vi "Lab Panel V5.23.vi"() -> ()   [LabVIEW 2013] (continued)
                n1762 = property on="SELECT LAB01-1" class="RadioBtnsControl (strict)"("DisabledEnum"=w3329) -> ()  [unwired: 2 in, 2 out]
                n1763 = property on="SELECT LAB01-2" class="RadioBtnsControl (strict)"("DisabledEnum"=w3328) -> ()  [unwired: 2 in, 2 out]
                n1764 = Not(x=w3338) -> (.not. x?=w3339:bool)
                n1765 = property on="RESULT LAB01-1" class="Bool (strict)"("Visible"=w3339) -> ()  [unwired: 2 in, 2 out]
                n1766 = Not(x=w3333) -> (.not. x?=w3337:bool)
                n1767 = Not(x=w3332) -> (.not. x?=w3336:bool)
                n1768 = Not(x=w3330) -> (.not. x?=w3335:bool)
                n1769 = property on="RESULT LAB01-2" class="Bool (strict)"("Visible"=w3337) -> ()  [unwired: 2 in, 2 out]
                n1770 = Not(x=w3331) -> (.not. x?=w3334:bool)
                n1771 = property on="RESULT LAB02-1" class="Bool (strict)"("Visible"=w3336) -> ()  [unwired: 2 in, 2 out]
                n1772 = property on="RESULT LAB02-2" class="Bool (strict)"("Visible"=w3335) -> ()  [unwired: 2 in, 2 out]
                n1773 = property on="RESULT LAB03-1" class="Bool (strict)"("Visible"=w3334) -> ()  [unwired: 2 in, 2 out]
                n1774 = property on="SET LAB01-1" class="Clust (strict)"("DisabledEnum"=w3329) -> ()  [unwired: 2 in, 2 out]
                n1775 = property on="SET LAB01-2" class="Clust (strict)"("DisabledEnum"=w3328) -> ()  [unwired: 2 in, 2 out]
                n1776 = property on="SET LAB02-1" class="Clust (strict)"("DisabledEnum"=w3327) -> ()  [unwired: 2 in, 2 out]
                n1777 = property on="SET LAB02-2" class="Clust (strict)"("DisabledEnum"=w3326) -> ()  [unwired: 2 in, 2 out]
                n1778 = property on="SET LAB03-1" class="Clust (strict)"("DisabledEnum"=w3325) -> ()  [unwired: 2 in, 2 out]
                n1779 = property on="O/I  LAB01-1" class="Bool (strict)"("DisabledEnum"=w3329) -> ()  [unwired: 2 in, 2 out]
                n1780 = property on="O/I  LAB01-2" class="Bool (strict)"("DisabledEnum"=w3328) -> ()  [unwired: 2 in, 2 out]
                n1781 = property on="O/I  LAB02-1" class="Bool (strict)"("DisabledEnum"=w3327) -> ()  [unwired: 2 in, 2 out]
                n1782 = property on="O/I  LAB02-2" class="Bool (strict)"("DisabledEnum"=w3326) -> ()  [unwired: 2 in, 2 out]
                n1783 = property on="O/I  LAB03-1" class="Bool (strict)"("DisabledEnum"=w3325) -> ()  [unwired: 2 in, 2 out]
              }
              frame #1 {
                n1784 = Select(t=2, s=w3359, f=0) -> (s? t:f=w3350:i32)
                n1785 = Select(t=2, s=w3358, f=0) -> (s? t:f=w3351:i32)
                n1786 = Select(t=2, s=w3355, f=0) -> (s? t:f=w3354:i32)
                n1787 = Select(t=2, s=w3356, f=0) -> (s? t:f=w3353:i32)
                n1788 = Select(t=2, s=w3357, f=0) -> (s? t:f=w3352:i32)
                n1789 = property on="SELECT LAB05-2" class="RadioBtnsControl (strict)"("DisabledEnum"=w3350) -> ()  [unwired: 2 in, 2 out]
                n1790 = property on="SELECT LAB05-1" class="RadioBtnsControl (strict)"("DisabledEnum"=w3351) -> ()  [unwired: 2 in, 2 out]
                n1791 = property on="SELECT LAB03-2" class="RadioBtnsControl (strict)"("DisabledEnum"=w3354) -> ()  [unwired: 2 in, 2 out]
                n1792 = property on="SELECT LAB04-1" class="RadioBtnsControl (strict)"("DisabledEnum"=w3353) -> ()  [unwired: 2 in, 2 out]
                n1793 = property on="SELECT LAB04-2" class="RadioBtnsControl (strict)"("DisabledEnum"=w3352) -> ()  [unwired: 2 in, 2 out]
                n1794 = property on="SET LAB05-2" class="Clust (strict)"("DisabledEnum"=w3350) -> ()  [unwired: 2 in, 2 out]
                n1795 = property on="SET LAB05-1" class="Clust (strict)"("DisabledEnum"=w3351) -> ()  [unwired: 2 in, 2 out]
                n1796 = property on="SET LAB03-2" class="Clust (strict)"("DisabledEnum"=w3354) -> ()  [unwired: 2 in, 2 out]
                n1797 = property on="SET LAB04-1" class="Clust (strict)"("DisabledEnum"=w3353) -> ()  [unwired: 2 in, 2 out]
                n1798 = property on="SET LAB04-2" class="Clust (strict)"("DisabledEnum"=w3352) -> ()  [unwired: 2 in, 2 out]
                n1799 = property on="O/I  LAB05-2" class="Bool (strict)"("DisabledEnum"=w3350) -> ()  [unwired: 2 in, 2 out]
                n1800 = property on="O/I  LAB05-1" class="Bool (strict)"("DisabledEnum"=w3351) -> ()  [unwired: 2 in, 2 out]
                n1801 = property on="O/I  LAB04-1" class="Bool (strict)"("DisabledEnum"=w3353) -> ()  [unwired: 2 in, 2 out]
                n1802 = property on="O/I  LAB04-2" class="Bool (strict)"("DisabledEnum"=w3352) -> ()  [unwired: 2 in, 2 out]
                n1803 = property on="O/I  LAB03-2" class="Bool (strict)"("DisabledEnum"=w3354) -> ()  [unwired: 2 in, 2 out]
                n1804 = Not(x=w3359) -> (.not. x?=w3360:bool)
                n1805 = Not(x=w3358) -> (.not. x?=w3361:bool)
                n1806 = Not(x=w3357) -> (.not. x?=w3362:bool)
                n1807 = property on="RESULT LAB05-2" class="Bool (strict)"("Visible"=w3360) -> ()  [unwired: 2 in, 2 out]
                n1808 = property on="RESULT LAB05-1" class="Bool (strict)"("Visible"=w3361) -> ()  [unwired: 2 in, 2 out]
                n1809 = Not(x=w3356) -> (.not. x?=w3363:bool)
                n1810 = property on="RESULT LAB04-2" class="Bool (strict)"("Visible"=w3362) -> ()  [unwired: 2 in, 2 out]
                n1811 = Not(x=w3355) -> (.not. x?=w3364:bool)
                n1812 = property on="RESULT LAB04-1" class="Bool (strict)"("Visible"=w3363) -> ()  [unwired: 2 in, 2 out]
                n1813 = property on="RESULT LAB03-2" class="Bool (strict)"("Visible"=w3364) -> ()  [unwired: 2 in, 2 out]
              }
              frame #2 {
                # "disable calibrate if any test running"
                n1814 = Or(x=w3387, y=w3386) -> (x .or. y?=w3380:bool)
                n1815 = Or(x=w3389, y=w3388) -> (x .or. y?=w3382:bool)
                n1816 = Or(x=w3393, y=w3392) -> (x .or. y?=w3384:bool)
                n1817 = Or(x=w3391, y=w3390) -> (x .or. y?=w3383:bool)
                n1818 = Or(x=w3395, y=w3394) -> (x .or. y?=w3385:bool)
                n1819 = Or(x=w3383, y=w3382) -> (x .or. y?=w3381:bool)
                n1820 = Or(x=w3385, y=w3384) -> (x .or. y?=w3379:bool)
                n1821 = Or(x=w3381, y=w3380) -> (x .or. y?=w3378:bool)
                n1822 = Or(x=w3379, y=w3378) -> (x .or. y?=w3377:bool)
                n1823 = case shown="False" w3377 {
                  tunnel: [0 2] -> w3376
                  frame False {
                  }
                  frame True {
                  }
                }
                n1824 = property on="JIG TEST" class="Clust (strict)"("DisabledEnum"=w3376) -> ()  [unwired: 2 in, 2 out]
                n1825 = property on="Network Directory" class="Path"("DisabledEnum"=w3376) -> ()  [unwired: 2 in, 2 out]
                n1826 = property on="MAIL SETTINGS" class="Clust (strict)"("DisabledEnum"=w3376) -> ()  [unwired: 2 in, 2 out]
                n1827 = property on="SET (cal)" class="Bool (strict)"("DisabledEnum"=w3376) -> ()  [unwired: 2 in, 2 out]
                n1828 = property on="ADMIN" class="Bool (strict)"("DisabledEnum"=0) -> ()  [unwired: 2 in, 2 out]
              }
            }
          }
          frame #8 {
            # "drive jigs"
            n1829 = stacked-sequence {
              frame #0 {
                # "jig on"
                n1830 = local read "jig cycle"() -> (w3403:dbl)
                n1831 = property on="JIG TEST" class="Clust (strict)"() -> ("DisabledEnum"=w3400:T16)  [unwired: 2 in, 2 out]
                n1832 = Equal?(x=w3400, y=2) -> (x = y?=w3399:bool)
                n1833 = Equal?(x=w3403, y=0) -> (x = y?=w3401:bool)
                n1834 = And(x=w3401, y=w3399) -> (x .and. y?=w3398:bool)
                n1835 = case shown="True" w3398 {
                  frame False {
                  }
                  frame True {
                    n1836 = local read "run lab01-1"() -> (w3414:bool)
                    n1837 = local read "run lab01-2"() -> (w3413:bool)
                    n1838 = local read "run lab02-1"() -> (w3412:bool)
                    n1839 = local read "run lab02-2"() -> (w3411:bool)
                    n1840 = local read "run lab03-1"() -> (w3410:bool)
                    n1841 = local read "run lab03-2"() -> (w3409:bool)
                    n1842 = local read "run lab04-1"() -> (w3408:bool)
                    n1843 = local read "run lab04-2"() -> (w3407:bool)
                    n1844 = local read "run lab05-1"() -> (w3406:bool)
                    n1845 = local read "run lab05-2"() -> (w3405:bool)
                    n1846 = local write "JIG LAB03-2"(w3409) -> ()
                    n1847 = local write "JIG LAB01-1"(w3414) -> ()
                    n1848 = local write "JIG LAB01-2"(w3413) -> ()
                    n1849 = local write "JIG LAB02-1"(w3412) -> ()
                    n1850 = local write "JIG LAB02-2"(w3411) -> ()
                    n1851 = local write "JIG LAB03-1"(w3410) -> ()
                    n1852 = local write "JIG LAB04-1"(w3408) -> ()
                    n1853 = local write "JIG LAB04-2"(w3407) -> ()
                    n1854 = local write "JIG LAB05-1"(w3406) -> ()
                    n1855 = local write "JIG LAB05-2"(w3405) -> ()
                  }
                }
              }
              frame #1 {
                # "jig off"
                n1856 = local read "jig cycle"() -> (w3421:dbl)
                n1857 = local read "on loops"() -> (w3420:dbl)
                n1858 = property on="JIG TEST" class="Clust (strict)"() -> ("DisabledEnum"=w3419:T16)  [unwired: 2 in, 2 out]
                n1859 = Equal?(x=w3419, y=2) -> (x = y?=w3417:bool)
                n1860 = Equal?(x=w3421, y=w3420) -> (x = y?=w3416:bool)
                n1861 = And(x=w3416, y=w3417) -> (x .and. y?=w3415:bool)
                n1862 = case shown="True" w3415 {
                  frame False {
                  }
                  frame True {
                    w3472 = FALSE
                    w3473 = TRUE
                    w3471 = 2
                    n1863 = local read "SELECT LAB05-2"() -> (w3462:T3)
                    n1864 = local read "SELECT LAB04-2"() -> (w3464:T3)
                    n1865 = local read "SELECT LAB04-1"() -> (w3465:T3)
                    n1866 = local read "SELECT LAB05-1"() -> (w3463:T3)
                    n1867 = local read "SELECT LAB03-2"() -> (w3466:T3)
                    n1868 = local read "SELECT LAB02-1"() -> (w3469:T3)
                    n1869 = local read "SELECT LAB03-1"() -> (w3467:T3)
                    n1870 = local read "SELECT LAB02-2"() -> (w3468:T3)
                    n1871 = local read "SELECT LAB01-2"() -> (w3470:T3)
                    n1872 = local read "run lab05-1"() -> (w3432:bool)
                    n1873 = local read "run lab05-2"() -> (w3431:bool)
                    n1874 = local read "SELECT LAB01-1"() -> (w3474:T3)
                    n1875 = local read "run lab04-2"() -> (w3433:bool)
                    n1876 = local read "run lab04-1"() -> (w3434:bool)
                    n1877 = local read "run lab01-1"() -> (w3450:bool)
                    n1878 = local read "run lab01-2"() -> (w3439:bool)
                    n1879 = local read "run lab03-2"() -> (w3435:bool)
                    n1880 = local read "run lab03-1"() -> (w3436:bool)
                    n1881 = local read "run lab02-1"() -> (w3438:bool)
                    n1882 = local read "run lab02-2"() -> (w3437:bool)
                    n1883 = Equal?(x=w3471, y=w3467) -> (x = y?=w3445:bool)
                    n1884 = Equal?(x=w3471, y=w3466) -> (x = y?=w3444:bool)
                    n1885 = Equal?(x=w3471, y=w3465) -> (x = y?=w3443:bool)
                    n1886 = Equal?(x=w3471, y=w3464) -> (x = y?=w3442:bool)
                    n1887 = Equal?(x=w3471, y=w3463) -> (x = y?=w3441:bool)
                    n1888 = Equal?(x=w3471, y=w3462) -> (x = y?=w3440:bool)
                    n1889 = Equal?(x=w3471, y=w3474) -> (x = y?=w3451:bool)
                    n1890 = Equal?(x=w3471, y=w3469) -> (x = y?=w3447:bool)
                    n1891 = Equal?(x=w3471, y=w3468) -> (x = y?=w3446:bool)
                    n1892 = Equal?(x=w3471, y=w3470) -> (x = y?=w3448:bool)
                    n1893 = And(x=w3442, y=w3433) -> (x .and. y?=w3424:bool)
                    n1894 = And(x=w3445, y=w3436) -> (x .and. y?=w3427:bool)
                    n1895 = And(x=w3443, y=w3434) -> (x .and. y?=w3425:bool)
                    n1896 = And(x=w3440, y=w3431) -> (x .and. y?=w3422:bool)
                    n1897 = And(x=w3446, y=w3437) -> (x .and. y?=w3428:bool)
                    n1898 = And(x=w3444, y=w3435) -> (x .and. y?=w3426:bool)
                    n1899 = And(x=w3441, y=w3432) -> (x .and. y?=w3423:bool)
                    n1900 = And(x=w3448, y=w3439) -> (x .and. y?=w3430:bool)
                    n1901 = And(x=w3451, y=w3450) -> (x .and. y?=w3449:bool)
                    n1902 = And(x=w3447, y=w3438) -> (x .and. y?=w3429:bool)
                    n1903 = Select(t=w3473, s=w3449, f=w3472) -> (s? t:f=w3452:bool)
                    n1904 = Select(t=w3473, s=w3430, f=w3472) -> (s? t:f=w3453:bool)
                    n1905 = Select(t=w3473, s=w3429, f=w3472) -> (s? t:f=w3454:bool)
                    n1906 = Select(t=w3473, s=w3428, f=w3472) -> (s? t:f=w3455:bool)
                    n1907 = Select(t=w3473, s=w3427, f=w3472) -> (s? t:f=w3456:bool)
                    n1908 = Select(t=w3473, s=w3426, f=w3472) -> (s? t:f=w3457:bool)
                    n1909 = Select(t=w3473, s=w3425, f=w3472) -> (s? t:f=w3458:bool)
                    n1910 = Select(t=w3473, s=w3424, f=w3472) -> (s? t:f=w3459:bool)
                    n1911 = Select(t=w3473, s=w3423, f=w3472) -> (s? t:f=w3460:bool)
                    n1912 = Select(t=w3473, s=w3422, f=w3472) -> (s? t:f=w3461:bool)
                    n1913 = local write "JIG LAB03-2"(w3457) -> ()
                    n1914 = local write "JIG LAB02-1"(w3454) -> ()
                    n1915 = local write "JIG LAB02-2"(w3455) -> ()
                    n1916 = local write "JIG LAB01-2"(w3453) -> ()
                    n1917 = local write "JIG LAB03-1"(w3456) -> ()
                    n1918 = local write "JIG LAB01-1"(w3452) -> ()
                    n1919 = local write "JIG LAB05-2"(w3461) -> ()
                    n1920 = local write "JIG LAB04-1"(w3458) -> ()
                    n1921 = local write "JIG LAB05-1"(w3460) -> ()
                    n1922 = local write "JIG LAB04-2"(w3459) -> ()
                  }
                }
              }
            }
          }
          frame #9 {
            # "enable  jig test output if no test busy"
            n1923 = property on="JIG TEST" class="Clust (strict)"() -> ("DisabledEnum"=w3477:T16)  [unwired: 2 in, 2 out]
            n1924 = Equal?(x=w3477, y=0) -> (x = y?=w3475:bool)
            n1925 = case shown="True" w3475 {
              frame False {
              }
              frame True {
                n1926 = local read "JIG TEST"() -> (w3488:T10)
                n1927 = Unbundle(w3488) -> ("LAB01-1"=w3487:bool, "LAB01-2"=w3486:bool, "LAB02-1"=w3485:bool, "LAB02-2"=w3484:bool, "LAB03-1"=w3483:bool, "LAB03-2"=w3482:bool, "LAB04-1"=w3481:bool, "LAB04-2"=w3480:bool, "LAB05-1"=w3479:bool, "LAB05-2"=w3478:bool)
                n1928 = local write "JIG LAB05-1"(w3479) -> ()
                n1929 = local write "JIG LAB05-2"(w3478) -> ()
                n1930 = local write "JIG LAB04-1"(w3481) -> ()
                n1931 = local write "JIG LAB04-2"(w3480) -> ()
                n1932 = local write "JIG LAB03-2"(w3482) -> ()
                n1933 = local write "JIG LAB01-1"(w3487) -> ()
                n1934 = local write "JIG LAB02-1"(w3485) -> ()
                n1935 = local write "JIG LAB03-1"(w3483) -> ()
                n1936 = local write "JIG LAB01-2"(w3486) -> ()
                n1937 = local write "JIG LAB02-2"(w3484) -> ()
              }
            }
          }
          frame #10 {
            w3490 = FALSE
            # "Drive digital output and reset USB and temperature network if required."
            n1938 = global read "Global display 3.vi" "cycle O/F"() -> (w3499:bool)
            n1939 = local read "O/I  LAB05-2"() -> (w3492:bool)
            n1940 = local read "O/I  LAB05-1"() -> (w3494:bool)
            n1941 = local read "JIG LAB05-2"() -> (w3491:bool)
            n1942 = local read "O/I  LAB04-2"() -> (w3496:bool)
            n1943 = local read "JIG LAB05-1"() -> (w3493:bool)
            n1944 = local read "JIG LAB04-2"() -> (w3495:bool)
            n1945 = local read "O/I  LAB03-1"() -> (w3510:bool)
            n1946 = local read "O/I  LAB04-1"() -> (w3506:bool)
            n1947 = local read "O/I  LAB02-1"() -> (w3514:bool)
            n1948 = local read "O/I  LAB02-2"() -> (w3512:bool)
            n1949 = local read "O/I  LAB03-2"() -> (w3508:bool)
            n1950 = local read "JIG LAB04-1"() -> (w3505:bool)
            n1951 = local read "JIG LAB03-2"() -> (w3507:bool)
            n1952 = local read "O/I  LAB01-2"() -> (w3516:bool)
            n1953 = local read "JIG LAB02-1"() -> (w3513:bool)
            n1954 = local read "JIG LAB02-2"() -> (w3511:bool)
            n1955 = local read "JIG LAB03-1"() -> (w3509:bool)
            n1956 = local read "O/I  LAB01-1"() -> (w3518:bool)
            n1957 = local read "JIG LAB01-2"() -> (w3515:bool)
            n1958 = local read "JIG LAB01-1"() -> (w3517:bool)
            n1959 = case shown="False" w3499 {
              tunnel: [w3644 w3647] -> w3498
              tunnel: [w3643 w3647] -> w3489
              frame False {
                n1960 = local read "Analog error"() -> (w3646:bool)
                n1961 = local read "Reset Measuring"() -> (w3645:bool)
                n1962 = local read "Error Temp"() -> (w3643:bool)
                n1963 = Or(x=w3645, y=w3646) -> (x .or. y?=w3644:bool)
              }
              frame True {
                w3647 = FALSE
              }
            }
            n1964 = Build Array(w3511, w3510, w3509, w3508, w3507, w3506, w3505) -> (w3503:bool[])
            n1965 = Build Array(w3518, w3517, w3516, w3515, w3514, w3513, w3512) -> (w3504:bool[])
            n1966 = Build Array(w3496, w3495, w3494, w3493, w3492, w3491, w3490, w3490) -> (w3502:bool[])
            n1967 = Not(x=w3499) -> (.not. x?=w3500:bool)
            n1968 = local read "Simulate"() -> (w3501:bool)
            n1969 = And(x=w3500, y=w3498) -> (x .and. y?=w3497:bool)
            n1970 = stacked-sequence {
              tunnel: w3504 -> [w3522 w3528 w3623]
              tunnel: w3503 -> [w3521 w3527 w3622]
              tunnel: w3502 -> [w3520 w3526 w3621]
              tunnel: w3501 -> [w3519 w3529 _]
              tunnel: w3497 -> [_ w3530 _]
              tunnel: w3489 -> [_ _ w3624]
              frame #0 {
                # "drive outputs for normal use"
                n1971 = case shown="False" w3519 {
                  tunnel: w3522 -> [w3525 _]
                  tunnel: w3521 -> [w3524 _]
                  tunnel: w3520 -> [w3523 _]
                  frame False {
                    n1972 = call "sub vi - Drive Relays All v6.vi"("Array #2"=w3523, "Array #1"=w3524, "Array #0"=w3525) -> ()  [unwired: 8 in, 1 out]
                  }
                  frame True {
                  }
                }
              }
              frame #1 {
                # "USB  reset routine"
                n1973 = case shown="True" w3530 {
                  tunnel: w3529 -> [_ w3534]
                  tunnel: w3528 -> [_ w3533]
                  tunnel: w3527 -> [_ w3532]
                  tunnel: w3526 -> [_ w3531]
                  frame False {
                  }
                  frame True {
                    n1974 = stacked-sequence {
                      seq-local: [w3536 _ _ _ _] -> [_ w3542 _ _ _]
                      tunnel: w3534 -> [_ w3546 _ _ _]
                      tunnel: w3533 -> [_ w3545 _ _ _]
                      tunnel: w3532 -> [_ w3544 _ _ _]
                      tunnel: w3531 -> [_ w3543 _ _ _]
                      frame #0 {
                        n1975 = case shown="False" "Auto Reset" {
                          tunnel: [w3539 FALSE] -> w3537
                          frame False {
                            n1976 = Two Button Dialog(message="System reset") -> (T button?=w3539:bool)  [unwired: 2 in]
                          }
                          frame True {
                          }
                        }
                        n1977 = disable-structure shown="Disabled" {
                          frame Disabled {
                            n1978 = local write "Tab Control 2"(5) -> ()
                          }
                          frame Enabled {
                          }
                        }
                        n1979 = Or(x="Auto Reset", y=w3537) -> (x .or. y?=w3536:bool)
                      }
                      frame #1 {
                        n1980 = case shown="True" w3542 {
                          tunnel: w3546 -> [_ w3552]
                          tunnel: w3545 -> [_ w3551]
                          tunnel: w3544 -> [_ w3550]
                          tunnel: w3543 -> [_ w3549]
                          frame False {
                          }
                          frame True {
                            n1981 = stacked-sequence {
                              tunnel: w3552 -> [_ w3570 _]
                              tunnel: bool[] [] -> [w3555 w3569 w3579]
                              tunnel: w3551 -> [_ _ w3578]
                              tunnel: w3550 -> [w3554 _ w3577]
                              tunnel: w3549 -> [w3553 _ w3576]
                              tunnel: 3000 -> [w3556 _ w3575]
                              frame #0 {
                                # "switch off test stations for system reset"
                                n1982 = stacked-sequence {
                                tunnel: w3556 -> [w3560 w3564 w3566]
                                tunnel: w3555 -> [w3559 w3563 w3567]
                                tunnel: w3554 -> [w3558 _ _]
                                tunnel: w3553 -> [w3557 w3562 _]
                                frame #0 {
                                # "drive 1st 7 inputs"
                                n1983 = call "sub vi - Drive Relays All v6.vi"("Array #2"=w3557, "Array #1"=w3558, "Array #0"=w3559) -> ()  [unwired: 8 in, 1 out]
                                n1984 = call "Message Display V1.vi"("Message"="Delay off LAB 01-1 to 02-1", "Delay mS"=w3560) -> ()  [unwired: 10 in]
                                }
                                frame #1 {
                                # "drive 2nd 7 inputs"
                                n1985 = call "sub vi - Drive Relays All v6.vi"("Array #2"=w3562, "Array #1"=w3563, "Array #0"=w3563) -> ()  [unwired: 8 in, 1 out]
                                n1986 = call "Message Display V1.vi"("Message"="Delay off LAB 02-2 to 04-1", "Delay mS"=w3564) -> ()  [unwired: 10 in]
                                }
                                frame #2 {
                                # "drive 3rd 7 inputs"
                                n1987 = call "sub vi - Drive Relays All v6.vi"("Array #2"=w3567, "Array #1"=w3567, "Array #0"=w3567) -> ()  [unwired: 8 in, 1 out]
                                n1988 = call "Message Display V1.vi"("Message"="Delay off LAB 04-2 to 05-2", "Delay mS"=w3566) -> ()  [unwired: 10 in]
                                }
                                }
                              }
                              frame #1 {
                                # "reset all usb modules"
                                n1989 = stacked-sequence {
                                tunnel: w3570 -> [_ w3574]
                                tunnel: w3569 -> [w3572 _]
                                frame #0 {
                                n1990 = call "sub vi - Drive Relays All v6.vi"("Array #2"=bool[] [FALSE, FALSE, FALSE, FALSE, FALSE, FALSE, TRUE, FALSE], "Array #1"=w3572, "Array #0"=w3572) -> ()  [unwired: 8 in, 1 out]
                                }
                                frame #1 {
                                n1991 = call "Reset Meas v 4.vi"("simulate"=w3574) -> ("Reset Error"=→"Reset Error":bool)  [unwired: 10 in]
                                }
                                }
                              }
                              frame #2 {
                                # "switch test stations back on after reset"
                                n1992 = stacked-sequence {
                                tunnel: w3579 -> [w3583 w3586 _]
                                tunnel: w3578 -> [w3582 w3588 w3593]
                                tunnel: w3575 -> [w3581 w3584 w3590]
                                tunnel: w3577 -> [_ w3587 w3592]
                                tunnel: w3576 -> [_ _ w3589]
                                frame #0 {
                                # "drive 1st 7 inputs"
                                n1993 = call "sub vi - Drive Relays All v6.vi"("Array #2"=w3583, "Array #1"=w3583, "Array #0"=w3582) -> ()  [unwired: 8 in, 1 out]
                                n1994 = call "Message Display V1.vi"("Message"="Delay on LAB 01-1 to 02-1", "Delay mS"=w3581) -> ()  [unwired: 10 in]
                                }
                                frame #1 {
                                # "drive 1st & 2nd outputs"
                                n1995 = call "sub vi - Drive Relays All v6.vi"("Array #2"=w3586, "Array #1"=w3587, "Array #0"=w3588) -> ()  [unwired: 8 in, 1 out]
                                n1996 = call "Message Display V1.vi"("Message"="Delay on LAB 02-2 to 04-1", "Delay mS"=w3584) -> ()  [unwired: 10 in]
                                }
                                frame #2 {
                                n1997 = call "sub vi - Drive Relays All v6.vi"("Array #2"=w3589, "Array #1"=w3592, "Array #0"=w3593) -> ()  [unwired: 8 in, 1 out]
                                n1998 = call "Message Display V1.vi"("Message"="Delay on LAB 04-2 to 05-2", "Delay mS"=w3590) -> ()  [unwired: 10 in]
                                }
                                }
                              }
                            }
                          }
                        }
                      }
                      frame #2 {
                        w3594 = 0
                        w3595 = FALSE
                        # "set all back to zero"
                        n1999 = local read "Total USB resets"() -> (w3597:dbl)
                        n2000 = local read "Resets Done"() -> (w3599:dbl)
                        n2001 = local write "Reset Measuring"(w3595) -> ()
                        n2002 = local write "Analog error"(w3595) -> ()
                        n2003 = local write "Er USB#2"(w3594) -> ()
                        n2004 = local write "Er USB#0"(w3594) -> ()
                        n2005 = local write "Er USB#1"(w3594) -> ()
                        n2006 = local write "Error USB #0"(w3595) -> ()
                        n2007 = local write "Error USB #1"(w3595) -> ()
                        n2008 = local write "Error USB #2"(w3595) -> ()
                        n2009 = Increment(x=w3597) -> (x+1=w3596:dbl)
                        n2010 = Increment(x=w3599) -> (x+1=→"Resets Done":dbl)
                        n2011 = local write "Total USB resets"(w3596) -> ()
                      }
                      frame #3 {
                        # "save reset value"
                        n2012 = String To Path(string="c:\\crabtree\\Set Up\\") -> (path=w3609:path)
                        n2013 = Build Path(base path=w3609, name or relative path="USB resets.bin") -> (appended path=w3602:path)
                        n2014 = Create Folder(path (use dialog)=w3609) -> (error out=w3601:errorcluster)  [unwired: 2 in, 2 out]
                        n2015 = local read "Total USB resets"() -> (w3600:dbl)
                        n2016 = call <vilib>:"Clear Errors.vi"("error in (no error)"=w3601) -> ()  [unwired: 6 in, 1 out]
                        n2017 = Open/Create/Replace File(file path (use dialog)=w3602, operation (0:open)=T17."replace or create") -> (refnum out=w3607:refnum<file>, error out=w3606:errorcluster)  [unwired: 4 in, 1 out]
                        n2018 = Write to Binary File(file (use dialog)=w3607, data=w3600, error in=w3606) -> (refnum out=w3605:refnum<file>, error out=w3604:errorcluster)  [unwired: 3 in, 1 out]
                        n2019 = Close File(refnum=w3605, error in=w3604) -> (error out=w3603:errorcluster)  [unwired: 1 out]
                        n2020 = local write "data file error"(w3603) -> ()
                      }
                      frame #4 {
                        # "mail reset value"
                        n2021 = local read "Total USB resets"() -> (w3617:dbl)
                        n2022 = local read "MAIL SETTINGS"() -> (w3613:T7)
                        n2023 = local read "Mail Test File To:"() -> (w3618:string)
                        n2024 = Number To Decimal String(number=w3617) -> (decimal integer string=w3615:string)  [unwired: 1 in]
                        n2025 = Unbundle(w3613) -> ("OUT SERVER ADDRESS"=w3620:string, "FROM ACCOUNT"=w3619:string)  [unwired: 5 out]
                        n2026 = Concatenate Strings("Total USB resets: ", w3615) -> (w3614:string)
                        n2027 = call "sub vi - send mail v5.vi"("TO:"=w3618, "subject"=w3614, "from"=w3619, "out going server"=w3620) -> ("error out"=w3612:errorcluster)  [unwired: 11 in]
                        n2028 = Bundle(cluster=w3613, "mail error"=w3612) -> ()  [unwired: 6 in, 1 out]
                      }
                    }
                  }
                }
              }
              frame #2 {
                # "reset temperature only"
                n2029 = case shown="True" w3624 {
                  tunnel: w3623 -> [_ w3627]
                  tunnel: w3622 -> [_ w3626]
                  tunnel: w3621 -> [_ w3625]
                  frame False {
                  }
                  frame True {
                    n2030 = stacked-sequence {
                      tunnel: w3627 -> [w3633 _ w3637 _]
                      tunnel: w3626 -> [w3632 _ w3636 _]
                      tunnel: w3625 -> [w3631 _ w3635 _]
                      frame #0 {
                        n2031 = Insert Into Array(array=w3631, index=7, new element=TRUE) -> (w3628:bool[])
                        n2032 = call "sub vi - Drive Relays All v6.vi"("Array #2"=w3628, "Array #1"=w3632, "Array #0"=w3633) -> ()  [unwired: 8 in, 1 out]
                      }
                      frame #1 {
                        n2033 = Wait (ms)(milliseconds to wait=500) -> ()  [unwired: 1 out]
                      }
                      frame #2 {
                        n2034 = Insert Into Array(array=w3635, index=7, new element=FALSE) -> (w3638:bool[])
                        n2035 = call "sub vi - Drive Relays All v6.vi"("Array #2"=w3638, "Array #1"=w3636, "Array #0"=w3637) -> ()  [unwired: 8 in, 1 out]
                      }
                      frame #3 {
                        w3642 = 0.0
                        n2036 = local write "Temp Er 04"(w3642) -> ()
                        n2037 = local write "Temp Er 02"(w3642) -> ()
                        n2038 = local write "Temp Er 01"(w3642) -> ()
                        n2039 = local write "Temp Er 03"(w3642) -> ()
                        n2040 = local write "Temp Er 05"(w3642) -> ()
                        n2041 = local write "Error Temp"(FALSE) -> ()
                      }
                    }
                  }
                }
              }
            }
          }
          frame #11 {
            # "get all analog values from USB devices"
            n2042 = local read "on loops"() -> (w3654:dbl)
            n2043 = local read "jig cycle"() -> (w3651:dbl)
            n2044 = Add(x=w3654, y=1) -> (x+y=w3652:dbl)
            n2045 = Equal?(x=w3651, y=1) -> (x = y?=w3648:bool)
            n2046 = Equal?(x=w3651, y=w3652) -> (x = y?=w3650:bool)
            n2047 = Or(x=w3648, y=w3650) -> (x .or. y?=w3649:bool)
            n2048 = global write "Global display 3.vi" "cycle O/F"(w3648) -> ()
            n2049 = case shown="True" w3649 {
              tunnel: w3648 -> [_ w3658]
              frame False {
              }
              frame True {
                n2050 = local read "Simulate"() -> (w3661:bool)
                n2051 = case shown="False" w3661 {
                  tunnel: [w3677 0.3 ("Analog loop time")] -> w3668
                  tunnel: [w3676 dynamicdata[] [] ("array GRAPH")] -> w3667
                  tunnel: [w3675 w3682] -> w3666
                  tunnel: [w3674 w3682] -> w3665
                  tunnel: [w3673 w3682] -> w3664
                  tunnel: [w3672 w3682] -> w3663
                  tunnel: [w3671 w3682] -> w3662
                  tunnel: w3658 -> [_ w3686]
                  tunnel: [w3670 "Ambient Volts"] -> w3657
                  tunnel: [w3669 bool[] []] -> w3656
                  frame False {
                    n2052 = call "sub vi - Read Analog All v9.3.vi"() -> ("Analog loop time"=w3677:dbl, "array GRAPH"=w3676:dynamicdata[], "LAB01"=w3675:T27, "LAB02"=w3674:T28, "LAB03"=w3673:T29, "LAB04"=w3672:T30, "deg C"=w3670:dbl, "USB Error"=w3669:bool[], "LAB05"=w3671:T31)  [unwired: 7 in]
                  }
                  frame True {
                    n2053 = local read "ON amps"() -> (w3680:dbl)
                    n2054 = local read "OFF amps"() -> (w3681:dbl)
                    n2055 = local read "VOLTS"() -> (w3684:dbl)
                    n2056 = local read "PF"() -> (w3683:dbl)
                    n2057 = Select(t=w3680, s=w3686, f=w3681) -> (s? t:f=w3685:dbl)
                    n2058 = Bundle("OFF amps"=w3685, "VOLTS"=w3684, "PF"=w3683, "OFF amps"=w3685, "VOLTS"=w3684, "PF"=w3683) -> (w3682:T32)  [unwired: 1 in]
                  }
                }
                n2059 = local read "Simulate"() -> (w3660:bool)
                n2060 = stacked-sequence {
                  seq-local: [w3691 _ _ _ _ _ _ _] -> [_ _ _ _ _ _ _ _]
                  seq-local: [w3690 _ _ _ _ _ _ _] -> [_ _ _ _ _ _ _ _]
                  seq-local: [w3689 _ _ _ _ _ _ _] -> [_ _ _ _ _ _ _ w3886]
                  tunnel: w3668 -> [_ w3744 _ _ _ _ _ _]
                  tunnel: w3667 -> [_ w3741 _ _ _ _ _ _]
                  tunnel: w3666 -> [_ _ w3771 _ _ _ _ _]
                  tunnel: w3665 -> [_ _ _ w3799 _ _ _ _]
                  tunnel: w3664 -> [_ _ _ _ w3827 _ _ _]
                  tunnel: w3663 -> [_ _ _ _ _ w3855 _ _]
                  tunnel: w3662 -> [_ _ _ _ _ _ w3883 _]
                  tunnel: w3660 -> [_ _ w3770 w3798 w3826 w3854 w3882 w3888]
                  tunnel: T14 {"1  (A) cal"=1.0, "1 (V) cal"=1.0, "1 (PF) cal"=1.0, "1 (TL) cal"=1.0, "1 (TN) cal"=1.0, "2 (A) cal"=1.0, "2 (V) cal"=1.0, "2 (PF) cal"=1.0, "2 (TL) cal"=1.0, "2 (TN) cal"=1.0} ("CAL LAB01") -> [_ _ w3769 w3797 w3825 w3853 w3881 _]
                  tunnel: w3657 -> [_ _ _ _ _ _ _ w3887]
                  tunnel: w3656 -> [w3694 _ _ _ _ _ _ _]
                  frame #0 {
                    n2061 = Index Array(array=w3694, index=2) -> (element=w3689:bool)
                    n2062 = Index Array(array=w3694, index=1) -> (element=w3690:bool)
                    n2063 = Index Array(array=w3694, index=0) -> (element=w3691:bool)
                    n2064 = local write "Error USB #2"(w3689) -> ()
                    n2065 = local write "Error USB #0"(w3691) -> ()
                    n2066 = local write "Error USB #1"(w3690) -> ()
                    n2067 = stacked-sequence {
                      tunnel: w3691 -> [w3698 _ _ _]
                      tunnel: w3690 -> [_ w3703 _ _]
                      tunnel: 0 -> [w3697 w3702 w3707 _]
                      tunnel: w3689 -> [_ _ w3708 _]
                      frame #0 {
                        n2068 = case shown="True" w3698 {
                          tunnel: w3697 -> [w3699 _]
                          frame False {
                            n2069 = local write "Er USB#0"(w3699) -> ()
                          }
                          frame True {
                            n2070 = local read "Er USB#0"() -> (w3701:dbl)
                            n2071 = Increment(x=w3701) -> (x+1=→"Er USB#0":dbl)
                          }
                        }
                      }
                      frame #1 {
                        n2072 = case shown="True" w3703 {
                          tunnel: w3702 -> [w3704 _]
                          frame False {
                            n2073 = local write "Er USB#1"(w3704) -> ()
                          }
                          frame True {
                            n2074 = local read "Er USB#1"() -> (w3706:dbl)
                            n2075 = Increment(x=w3706) -> (x+1=→"Er USB#1":dbl)
                          }
                        }
                      }
                      frame #2 {
                        n2076 = case shown="True" w3708 {
                          tunnel: w3707 -> [w3709 _]
                          frame False {
                            n2077 = local write "Er USB#2"(w3709) -> ()
                          }
                          frame True {
                            n2078 = local read "Er USB#2"() -> (w3711:dbl)
                            n2079 = Increment(x=w3711) -> (x+1=→"Er USB#2":dbl)
                          }
                        }
                      }
                      frame #3 {
                        w3717 = 5
                        n2080 = local read "Er USB#2"() -> (w3718:dbl)
                        n2081 = local read "Er USB#0"() -> (w3720:dbl)
                        n2082 = local read "Er USB#1"() -> (w3719:dbl)
                        n2083 = Greater Or Equal?(x=w3720, y=w3717) -> (x >= y?=w3715:bool)
                        n2084 = Greater Or Equal?(x=w3719, y=w3717) -> (x >= y?=w3714:bool)
                        n2085 = Greater Or Equal?(x=w3718, y=w3717) -> (x >= y?=w3713:bool)
                        n2086 = Or(x=w3715, y=w3714) -> (x .or. y?=w3716:bool)
                        n2087 = Or(x=w3716, y=w3713) -> (x .or. y?=→"Analog error":bool)
                      }
                    }
                  }
                  frame #1 {
                    # "display graph data on ADM page"
                    n2088 = local write "AI"(TRUE) -> ()
                    n2089 = global write "Global 1.vi" "RATE(Hz)"("RATE (Hz)") -> ()
                    n2090 = global write "Global 1.vi" "SAMPLES"("SAMPLES") -> ()
                    n2091 = Index Array(array=w3741, index=6) -> (element=→"LAB04-1 (GRAPH)":dynamicdata)
                    n2092 = Index Array(array=w3741, index=7) -> (element=→"LAB04-2 (GRAPH)":dynamicdata)
                    n2093 = Index Array(array=w3741, index=9) -> (element=→"LAB05-2 (GRAPH)":dynamicdata)
                    n2094 = Index Array(array=w3741, index=8) -> (element=→"LAB05-1 (GRAPH)":dynamicdata)
                    n2095 = Index Array(array=w3741, index=5) -> (element=→"LAB03-2 (GRAPH)":dynamicdata)
                    n2096 = Index Array(array=w3741, index=0) -> (element=→"LAB01-1 (GRAPH)":dynamicdata)
                    n2097 = Index Array(array=w3741, index=1) -> (element=→"LAB01-2 (GRAPH)":dynamicdata)
                    n2098 = Index Array(array=w3741, index=2) -> (element=→"LAB02-1 (GRAPH)":dynamicdata)
                    n2099 = Index Array(array=w3741, index=3) -> (element=→"LAB02-2 (GRAPH)":dynamicdata)
                    n2100 = Index Array(array=w3741, index=4) -> (element=→"LAB03-1 (GRAPH)":dynamicdata)
                    "AI loop time" <- w3744
                  }
                  frame #2 {
                    n2101 = case shown="False" w3770 {
                      tunnel: [w3772 w3773] -> w3768
                      tunnel: w3769 -> [_ w3773]
                      frame False {
                        n2102 = local read "CAL LAB01"() -> (w3772:T14)
                      }
                      frame True {
                      }
                    }
                    n2103 = Unbundle By Name(w3771) -> ("OFF amps"=w3767:dbl, "VOLTS"=w3766:dbl, "PF"=w3765:dbl, "OFF amps"=w3764:dbl, "VOLTS"=w3763:dbl, "PF"=w3762:dbl)
                    n2104 = Unbundle By Name(w3768) -> ("1  (A) cal"=w3761:dbl, "1 (V) cal"=w3760:dbl, "1 (PF) cal"=w3759:dbl, "2 (A) cal"=w3758:dbl, "2 (V) cal"=w3757:dbl, "2 (PF) cal"=w3756:dbl)  [unwired: 4 out]
                    n2105 = Multiply(x=w3767, y=w3761) -> (x*y=w3754:dbl)
                    n2106 = Multiply(x=w3766, y=w3760) -> (x*y=w3753:dbl)
                    n2107 = Multiply(x=w3765, y=w3759) -> (x*y=w3752:dbl)
                    n2108 = Multiply(x=w3764, y=w3758) -> (x*y=w3750:dbl)
                    n2109 = Multiply(x=w3763, y=w3757) -> (x*y=w3749:dbl)
                    n2110 = Multiply(x=w3762, y=w3756) -> (x*y=w3748:dbl)
                    n2111 = local read "SIG LAB01-1"() -> (w3755:T2)
                    n2112 = local read "SIG LAB01-2"() -> (w3751:T2)
                    n2113 = Bundle By Name(cluster=w3755, "AMPS"=w3754, "VOLTS"=w3753, "PF"=w3752) -> (w3747:T2)
                    n2114 = Bundle By Name(cluster=w3751, "AMPS"=w3750, "VOLTS"=w3749, "PF"=w3748) -> (w3746:T2)
                    n2115 = global write "Global display 1.vi" "SIG LAB01-2"(w3746) -> ()
                    n2116 = global write "Global display 1.vi" "SIG LAB01-1"(w3747) -> ()
                    n2117 = local write "SIG LAB01-2"(w3746) -> ()
                    n2118 = local write "SIG LAB01-1"(w3747) -> ()
                  }
                  frame #3 {
                    n2119 = Unbundle By Name(w3799) -> ("OFF amps"=w3795:dbl, "VOLTS"=w3794:dbl, "PF"=w3793:dbl, "OFF amps"=w3792:dbl, "VOLTS"=w3791:dbl, "PF"=w3790:dbl)
                    n2120 = case shown="True" w3798 {
                      tunnel: [w3800 w3801] -> w3796
                      tunnel: w3797 -> [_ w3801]
                      frame False {
                        n2121 = local read "CAL LAB02"() -> (w3800:T15)
                      }
                      frame True {
                      }
                    }
                    n2122 = Unbundle By Name(w3796) -> ("1  (A) cal"=w3789:dbl, "1 (V) cal"=w3788:dbl, "1 (PF) cal"=w3787:dbl, "2 (A) cal"=w3786:dbl, "2 (V) cal"=w3785:dbl, "2 (PF) cal"=w3784:dbl)  [unwired: 4 out]
                    n2123 = Multiply(x=w3795, y=w3789) -> (x*y=w3782:dbl)
                    n2124 = Multiply(x=w3794, y=w3788) -> (x*y=w3781:dbl)
                    n2125 = Multiply(x=w3793, y=w3787) -> (x*y=w3780:dbl)
                    n2126 = Multiply(x=w3792, y=w3786) -> (x*y=w3778:dbl)
                    n2127 = Multiply(x=w3791, y=w3785) -> (x*y=w3777:dbl)
                    n2128 = Multiply(x=w3790, y=w3784) -> (x*y=w3776:dbl)
                    n2129 = local read "SIG LAB02-1"() -> (w3783:T2)
                    n2130 = local read "SIG LAB02-2"() -> (w3779:T2)
                    n2131 = Bundle By Name(cluster=w3783, "AMPS"=w3782, "VOLTS"=w3781, "PF"=w3780) -> (w3775:T2)
                    n2132 = Bundle By Name(cluster=w3779, "AMPS"=w3778, "VOLTS"=w3777, "PF"=w3776) -> (w3774:T2)
                    n2133 = global write "Global display 1.vi" "SIG LAB02-1"(w3775) -> ()
                    n2134 = local write "SIG LAB02-2"(w3774) -> ()
                    n2135 = global write "Global display 1.vi" "SIG LAB02-2"(w3774) -> ()
                    n2136 = local write "SIG LAB02-1"(w3775) -> ()
                  }
                  frame #4 {
                    n2137 = Unbundle By Name(w3827) -> ("OFF amps"=w3823:dbl, "VOLTS"=w3822:dbl, "PF"=w3821:dbl, "OFF amps"=w3820:dbl, "VOLTS"=w3819:dbl, "PF"=w3818:dbl)
                    n2138 = case shown="True" w3826 {
                      tunnel: [w3828 w3829] -> w3824
                      tunnel: w3825 -> [_ w3829]
                      frame False {
                        n2139 = local read "CAL LAB03"() -> (w3828:T14)
                      }
                      frame True {
                      }
                    }
                    n2140 = Unbundle By Name(w3824) -> ("1  (A) cal"=w3817:dbl, "1 (V) cal"=w3816:dbl, "1 (PF) cal"=w3815:dbl, "2 (A) cal"=w3814:dbl, "2 (V) cal"=w3813:dbl, "2 (PF) cal"=w3812:dbl)  [unwired: 4 out]
                    n2141 = Multiply(x=w3823, y=w3817) -> (x*y=w3810:dbl)
                    n2142 = Multiply(x=w3822, y=w3816) -> (x*y=w3804:dbl)
                    n2143 = Multiply(x=w3821, y=w3815) -> (x*y=w3809:dbl)
                    n2144 = Multiply(x=w3820, y=w3814) -> (x*y=w3807:dbl)
                    n2145 = Multiply(x=w3819, y=w3813) -> (x*y=w3806:dbl)
                    n2146 = Multiply(x=w3818, y=w3812) -> (x*y=w3805:dbl)
                    n2147 = local read "SIG LAB03-1"() -> (w3811:T2)
                    n2148 = local read "SIG LAB03-2"() -> (w3808:T2)
                    n2149 = Bundle By Name(cluster=w3811, "AMPS"=w3810, "VOLTS"=w3804, "PF"=w3809) -> (w3803:T2)
                    n2150 = Bundle By Name(cluster=w3808, "AMPS"=w3807, "VOLTS"=w3806, "PF"=w3805) -> (w3802:T2)
                    n2151 = global write "Global display 1.vi" "SIG LAB03-1"(w3803) -> ()
                    n2152 = global write "Global display 1.vi" "SIG LAB03-2"(w3802) -> ()
                    n2153 = local write "SIG LAB03-2"(w3802) -> ()
                    n2154 = local write "SIG LAB03-1"(w3803) -> ()
                  }
                  frame #5 {
                    n2155 = case shown="False" w3854 {
                      tunnel: [w3856 w3857] -> w3852
                      tunnel: w3853 -> [_ w3857]
                      frame False {
                        n2156 = local read "CAL LAB04"() -> (w3856:T14)
                      }
                      frame True {
                      }
                    }
                    n2157 = Unbundle By Name(w3855) -> ("OFF amps"=w3851:dbl, "VOLTS"=w3850:dbl, "PF"=w3849:dbl, "OFF amps"=w3848:dbl, "VOLTS"=w3847:dbl, "PF"=w3846:dbl)
                    n2158 = Unbundle By Name(w3852) -> ("1  (A) cal"=w3845:dbl, "1 (V) cal"=w3844:dbl, "1 (PF) cal"=w3843:dbl, "2 (A) cal"=w3842:dbl, "2 (V) cal"=w3841:dbl, "2 (PF) cal"=w3840:dbl)  [unwired: 4 out]
                    n2159 = Multiply(x=w3851, y=w3845) -> (x*y=w3838:dbl)
                    n2160 = Multiply(x=w3850, y=w3844) -> (x*y=w3837:dbl)
                    n2161 = Multiply(x=w3849, y=w3843) -> (x*y=w3836:dbl)
                    n2162 = Multiply(x=w3848, y=w3842) -> (x*y=w3834:dbl)
                    n2163 = Multiply(x=w3847, y=w3841) -> (x*y=w3833:dbl)
                    n2164 = Multiply(x=w3846, y=w3840) -> (x*y=w3832:dbl)
                    n2165 = local read "SIG LAB04-1"() -> (w3839:T2)
                    n2166 = local read "SIG LAB04-2"() -> (w3835:T2)
                    n2167 = Bundle By Name(cluster=w3839, "AMPS"=w3838, "VOLTS"=w3837, "PF"=w3836) -> (w3831:T2)
                    n2168 = Bundle By Name(cluster=w3835, "AMPS"=w3834, "VOLTS"=w3833, "PF"=w3832) -> (w3830:T2)
                    n2169 = global write "Global display 1.vi" "SIG LAB04-2"(w3830) -> ()
                    n2170 = global write "Global display 1.vi" "SIG LAB04-1"(w3831) -> ()
                    n2171 = local write "SIG LAB04-2"(w3830) -> ()
                    n2172 = local write "SIG LAB04-1"(w3831) -> ()
                  }
                  frame #6 {
                    n2173 = Unbundle By Name(w3883) -> ("OFF amps"=w3879:dbl, "VOLTS"=w3860:dbl, "PF"=w3878:dbl, "OFF amps"=w3877:dbl, "VOLTS"=w3876:dbl, "PF"=w3875:dbl)
                    n2174 = case shown="False" w3882 {
                      tunnel: [w3884 w3885] -> w3880
                      tunnel: w3881 -> [_ w3885]
                      frame False {
                        n2175 = local read "CAL LAB05"() -> (w3884:T14)
                      }
                      frame True {
                      }
                    }
                    n2176 = Unbundle By Name(w3880) -> ("1  (A) cal"=w3874:dbl, "1 (V) cal"=w3873:dbl, "1 (PF) cal"=w3872:dbl, "2 (A) cal"=w3871:dbl, "2 (V) cal"=w3870:dbl, "2 (PF) cal"=w3869:dbl)  [unwired: 4 out]
                    n2177 = Multiply(x=w3879, y=w3874) -> (x*y=w3867:dbl)
                    n2178 = Multiply(x=w3860, y=w3873) -> (x*y=w3866:dbl)
                    n2179 = Multiply(x=w3878, y=w3872) -> (x*y=w3865:dbl)
                    n2180 = Multiply(x=w3877, y=w3871) -> (x*y=w3863:dbl)
                    n2181 = Multiply(x=w3876, y=w3870) -> (x*y=w3862:dbl)
                    n2182 = Multiply(x=w3875, y=w3869) -> (x*y=w3861:dbl)
                    n2183 = local read "SIG LAB05-1"() -> (w3868:T2)
                    n2184 = local read "SIG LAB05-2"() -> (w3864:T2)
                    n2185 = Bundle By Name(cluster=w3868, "AMPS"=w3867, "VOLTS"=w3866, "PF"=w3865) -> (w3859:T2)
                    n2186 = Bundle By Name(cluster=w3864, "AMPS"=w3863, "VOLTS"=w3862, "PF"=w3861) -> (w3858:T2)
                    n2187 = global write "Global display 1.vi" "SIG LAB05-1"(w3859) -> ()
                    n2188 = global write "Global display 1.vi" "SIG LAB05-2"(w3858) -> ()
                    n2189 = local write "SIG LAB05-2"(w3858) -> ()
                    n2190 = local write "SIG LAB05-1"(w3859) -> ()
                  }
                  frame #7 {
                    n2191 = case shown="False" w3886 {
                      tunnel: w3888 -> [w3890 _]
                      tunnel: w3887 -> [w3889 _]
                      frame False {
                        # "update ambient referance temperature"
                        n2192 = case shown="True" w3890 {
                          tunnel: [w3893 100.0] -> w3892
                          frame False {
                            n2193 = local read "TEMP REF cal"() -> (w3893:dbl)
                          }
                          frame True {
